vi "agilent_34970A_temperaures.vi"(3 "error in (no error)":errorcluster, 4 "TempProbeSet in":refnum<class "TempProbeSet.lvclass">, 5 "Readings":u16=1, 6 "Agilent Port In":refnum<visa-resource-name>="COM35") -> (0 "error out":errorcluster, 1 "TempProbeSet out":refnum<class "TempProbeSet.lvclass">, 2 "Agilent Port Out":refnum<visa-resource-name>="COM35")   [LabVIEW 2010]
uses:
  ProbeClass/TempProbeSet.lvclass
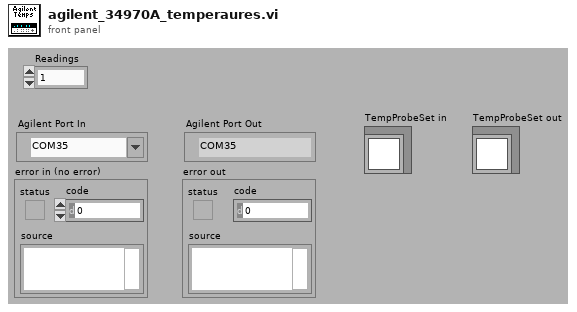
[diagram p1: front panel]
types:
  T1 = enum16{"Enable Register", "Event Register", "Operation Complete Bit"}
  T2 = enum16{"Manual", "Minimum", "Maximum", "Infinity"}
  T3 = enum16{"Bus", "Immediate", "External", "Alarm 1", "Alarm 2", "Alarm 3", "Alarm 4", "Timer"}
  T4 = cluster{"Include Alarm Data? (F:No)":bool, "Include Channel #? (F:No)":bool, "Include Time? (F:No)":bool, "Include Units? (F:No)":bool}
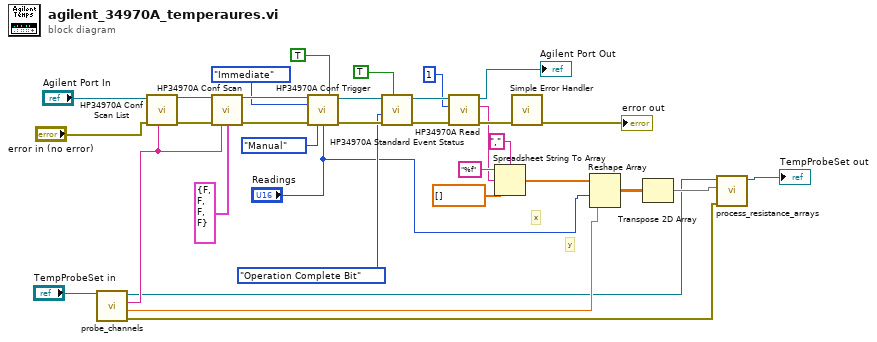
[diagram p0: block diagram]
diagram:
  # "y"
  # "x"
  n1 = call "probe_channels.vi"("TempProbeSet in"="TempProbeSet in") -> ("error out"=w2:errorcluster, "number of channels"=w6:dbl, "channels"=w7:string, "TempProbeSet out"=w3:refnum<class "TempProbeSet.lvclass">)  [unwired: 7 in]
  n2 = call "HP34970A Conf Scan List.vi"("Scan List (empty)"=w7, "error in (no error)"="error in (no error)", "VISA resource name"="Agilent Port In") -> ("error out"=w30:errorcluster, "VISA resource name out"=w31:refnum<visa-resource-name>)  [unwired: 6 in, 1 out]
  n3 = call "HP34970A Conf Scan.vi"("VISA resource name"=w31, "error in (no error)"=w30, "Channel List (empty)"=w7, "Scan Fields"=T4 {"Include Alarm Data? (F:No)"=FALSE, "Include Channel #? (F:No)"=FALSE, "Include Time? (F:No)"=FALSE, "Include Units? (F:No)"=FALSE}) -> ("VISA resource name out"=w28:refnum<visa-resource-name>, "error out"=w27:errorcluster)  [unwired: 9 in, 1 out]
  n4 = call "HP34970A Conf Trigger.vi"("VISA resource name"=w28, "Wait for Trigger? (F:No)"=TRUE, "Source (1:Immediate)"=T3."Immediate", "error in (no error)"=w27, "Max Trigger Count (3:Inf)"=T2."Manual", "# Triggers (1)"="Readings") -> ("VISA resource name out"=w23:refnum<visa-resource-name>, "error out"=w22:errorcluster)  [unwired: 7 in, 1 out]
  n5 = call "HP34970A Standard Event Status.vi"("Set/Check? (F:Set)"=TRUE, "error in (no error)"=w22, "Check Parameter (0:Enable Reg)"=T1."Operation Complete Bit", "VISA resource name"=w23) -> ("error out"=w33:errorcluster, "VISA resource name out"=w32:refnum<visa-resource-name>)  [unwired: 5 in, 1 out]
  n6 = call "HP34970A Read.vi"("error in (no error)"=w33, "# Channels (1)"=1, "VISA resource name"=w32) -> ("error out"=w34:errorcluster, "Readings"=w14:string, "VISA resource name out"=→"Agilent Port Out":refnum<visa-resource-name>)  [unwired: 5 in, 1 out]
  n7 = Spreadsheet String To Array(delimiter (Tab)=",", format string="%f", spreadsheet string=w14, array type (2D Dbl)=dbl[] []) -> (array=w9:dbl[])
  n8 = call <vilib>:"Simple Error Handler.vi"("error in (no error)"=w34) -> ("error out"=→"error out":errorcluster)  [unwired: 4 in, 4 out]
  n9 = Reshape Array(w9, "Readings", w6) -> (w10:dbl[][])
  n10 = Transpose 2D Array(2D array=w10) -> (transposed array=w4:dbl[][])
  n11 = call "process_resistance_arrays.vi"("error in (no error)"=w2, "Array"=w4, "TempProbeSet in"=w3) -> ("TempProbeSet out"=→"TempProbeSet out":refnum<class "TempProbeSet.lvclass">)  [unwired: 7 in, 1 out]
